vi "Read (Multiple Waveforms).vi"(8 "error in (no error)":errorcluster, 9 "Maximum Time (10000ms)":u32=10000, 10 "Channels":u16[](array[ring]) items=["Channel 1", "Channel 2", "Channel 3", "Channel 4", "Math", "Reference 1", "Reference 2", "Reference 3", "Reference 4", "D0", "D1", "D2", "D3", "D4", "D5", "D6", "D7", "D8", "D9", "D10", "D11", "D12", "D13", "D14", "D15", "Amplitude", "Frequency", "Phase", "Normal", "Average", "Maximum Peak Hold", "Minimum Peak Hold"], 11 "VISA resource name":refnum<visa-resource-name>) -> (0 "error out":errorcluster, 2 "Waveform Data":waveform(dbl)[](graph), 3 "VISA resource name out":refnum<visa-resource-name>)   [LabVIEW 2017, in "Scope.lvlib" / "Tektronix DPO MSO 2000 4000 Series.lvlib"]
doc: "Initiates an acquisition on all channels that you enabled with the <B>Configure Channel</B> VI. The VI waits for the acquisition to complete and returns the waveform for the <B>Channels</B> you specified. The <B>Timeout</B> control specifies the maximum time to wait for operation complete in milliseconds. If the oscilloscope did not complete the acquisition within the time period you specify with the Timeout parameter, the VI returns a timeout error. A common cause for a timeout error is the acquisition was not triggered. For example, the trigger level is out of range of the waveform."
uses:
  Tektronix DPO MSO 2000 4000 Series.lvlib
  Data_Low Level/RG Fetch Waveform (Waveform Data Type) with delay.vi
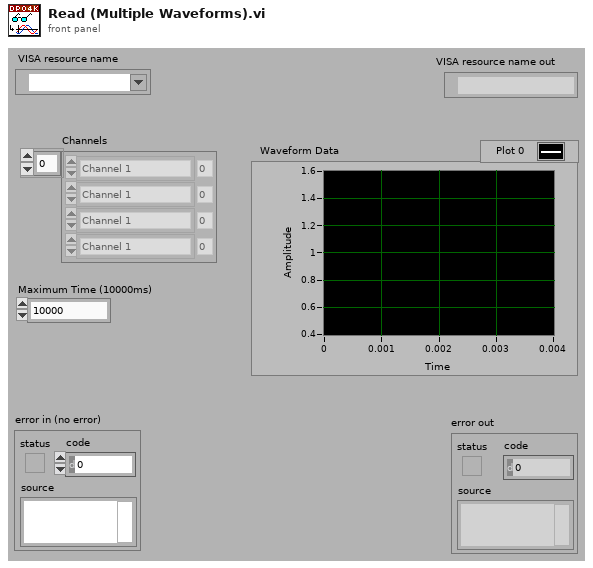
[diagram p1: front panel]
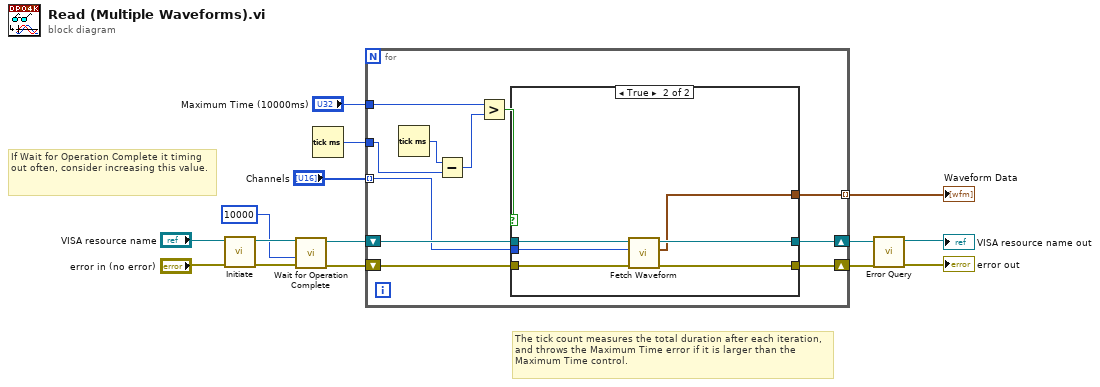
[diagram p0: block diagram]
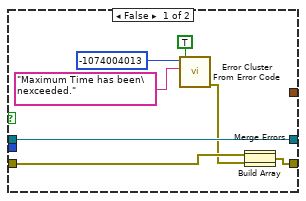
[diagram p2: hidden frame]
diagram:
  # "If Wait for Operation Complete it timing out often, consider increasing this value."
  # "The tick count measures the total duration after each iteration, and throws the Maximum Time error if it is larger than the Maximum Time control."
  n1 = call "Initiate.vi"("error in (no error)"="error in (no error)", "VISA resource name"="VISA resource name") -> ("error out"=w6:errorcluster, "VISA resource name out"=w7:refnum<visa-resource-name>)  [unwired: 8 in]
  n2 = call "Wait for Operation Complete.vi"("error in (no error)"=w6, "Maximum Time (10000ms)"=u32 10000, "VISA resource name"=w7) -> ("error out"=w4:errorcluster, "VISA resource name out"=w5:refnum<visa-resource-name>)  [unwired: 7 in]
  n3 = Tick Count (ms)() -> (millisecond timer value=w2:u32)
  n4 = for {
    shift-right: [w24] -> w14
    shift-left: w5 -> [w25]
    shift-right: [w23] -> w13
    shift-left: w4 -> [w26]
    tunnel: "Channels" -> [w22] mode=indexing
    tunnel: [w21] -> w10 mode=indexing
    tunnel: w2 -> [w19]
    tunnel: "Maximum Time (10000ms)" -> [w18]
    n5 = Tick Count (ms)() -> (millisecond timer value=w20:u32)
    n6 = Subtract(x=w20, y=w19) -> (x-y=w17:u32)
    n7 = Greater?(x=w18, y=w17) -> (0:w16:bool)
    n8 = case shown="True" w16 {
      tunnel: w26 -> [w29 w40]
      tunnel: w25 -> [w34 w39]
      tunnel: [w34 w38] -> w24
      tunnel: [w30 w37] -> w23
      tunnel: w22 -> [_ w36]
      tunnel: [_ w35] -> w21
      frame False {
        n9 = call <vilib>:"Error Cluster From Error Code.vi"("show call chain? (False)"=TRUE, "error message (\"\")"="Maximum Time has been\nexceeded." ("error message (\"\")"), "error code (0)"=-1074004013) -> ("error out"=w28:errorcluster)  [unwired: 6 in]
        n10 = Build Array(w29, w28) -> (w27:errorcluster[])
        n11 = Merge Errors(w27) -> (w30:errorcluster)
      }
      frame True {
        n12 = call-poly "Fetch Waveform.vi"("error in (no error)"=w40, "Channel (0: Channel 1)"=w36, "VISA resource name"=w39) -> ("error out"=w37:errorcluster, "Waveform Data"=w35:waveform(dbl), "VISA resource name out"=w38:refnum<visa-resource-name>)  [unwired: 6 in]
      }
    }
  }
  "Waveform Data" <- w10
  n13 = call "Error Query.vi"("error in (no error)"=w13, "VISA resource name"=w14) -> ("error out"=→"error out":errorcluster, "VISA resource name out"=→"VISA resource name out":refnum<visa-resource-name>)  [unwired: 6 in, 2 out]
